vi "429 RT Driver Init.vi"(8 "error in":errorcluster, 11 "Device Reference in":T1 format="%.0x") -> (0 "error out":errorcluster, 1 "tx channel handle array":u32[](array[numeric]), 2 "rx channel handle array":u32[](array[numeric]), 3 "Device Reference out":T1 format="%.0x", 5 "board handle":u32)   [LabVIEW 2016, in "Ballard Arinc-429 Engine.lvlib"]
uses:
  Ballard Arinc-429 Engine.lvlib
  <vilib>/NI Veristand/Custom Device API/Custom Device Item Ref.ctl
  Shared/Controls and Global/Specify module by.ctl
  <instrlib>/AIT 429/Private/AIT 429 Initialize (SlotID).vi
  <instrlib>/AIT 429/Private/AIT 429 Initialize (Index).vi
  <instrlib>/AIT 429/Private/AIT 429 Initialize (Serial Number).vi
  <vilib>/NI Veristand/Custom Device API/Get Item Property (Variant).vi
  <vilib>/NI Veristand/Custom Device API/Get Item Property (U16).vi
  <vilib>/NI Veristand/Custom Device API/Get Item Property (Path).vi
  Shared/Controls and Global/Global.vi
  <vilib>/NI Veristand/Custom Device API/Custom Device API.lvlib
  Shared/Ballard Arinc-429 Shared.lvlib
  <instrlib>/AIT 429/AIT 429.lvlib
  <userlib>/ARINC-429/Owl429.lvlib
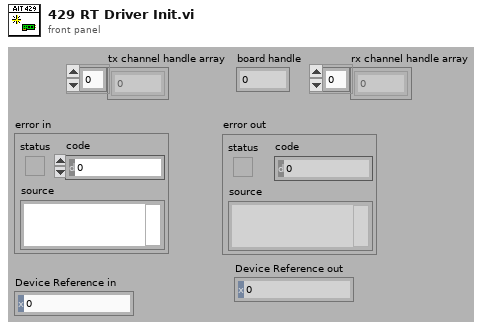
[diagram p1: front panel]
types:
  T1 = typedef "Custom Device API.lvlib/Custom Device Item Ref.ctl" = u64
  T2 = typedef "Ballard Arinc-429 Shared.lvlib/Specify module by.ctl" = enum16{"Index", "SlotID", "Serial number"}
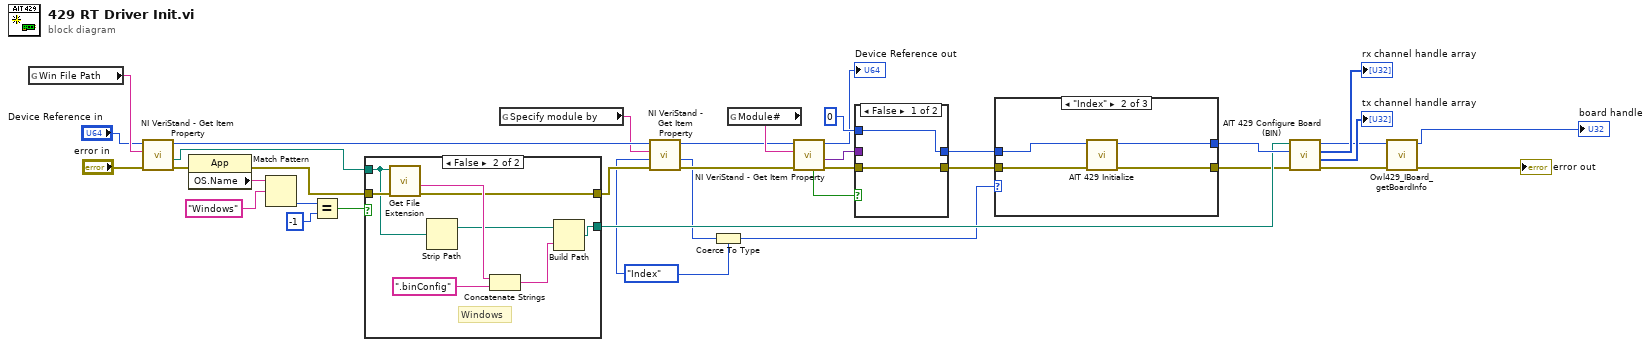
[diagram p0: block diagram]
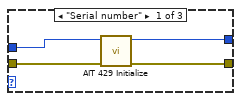
[diagram p2: hidden frame]
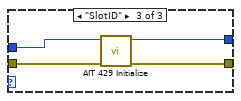
[diagram p3: hidden frame]
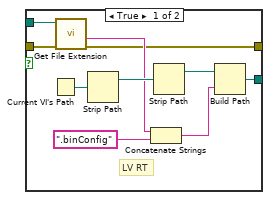
[diagram p4: hidden frame]
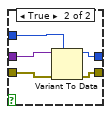
[diagram p5: hidden frame]
diagram:
  w3 = Specify_module_by."Index" ("Specify module by")
  n1 = global read "Global.vi" "Win File Path"() -> (w29:string)
  n2 = call-poly <vilib>:"NI VeriStand - Get Item Property.vi"("error in (no error)"="error in", "Property Name"=w29, "Item Ref in"="Device Reference in") -> ("error out"=w21:errorcluster, "Value"=w16:path, "Item Ref out"=w6:T1)  [unwired: 5 in, 1 out]
  n3 = property class="App"(error in=w21) -> (error out=w17:errorcluster, "OS.Name"=w10:string)  [unwired: 1 in, 1 out]
  n4 = Match Pattern(string=w10, regular expression="Windows") -> (offset past match=w19:i32)  [unwired: 1 in, 3 out]
  n5 = Equal?(x=w19, y=-1) -> (x = y?=w13:bool)
  n6 = case shown="False" w13 {
    tunnel: w17 -> [w37 w49]
    tunnel: w16 -> [w40 w48]
    tunnel: [w39 w51] -> w15
    tunnel: [w38 w50] -> w14
    frame True {
      # "LV RT"
      n7 = Current VI's Path() -> (path=w42:path)
      n8 = call <vilib>:"Get File Extension.vi"("error in (no error)"=w37, "file"=w40) -> ("error out"=w39:errorcluster, "filename without extension"=w41:string)  [unwired: 5 in, 3 out]
      n9 = Strip Path(path=w42) -> (stripped path=w43:path)  [unwired: 1 out]
      n10 = Concatenate Strings(w41, ".binConfig" ("string")) -> (w45:string)
      n11 = Strip Path(path=w43) -> (stripped path=w44:path)  [unwired: 1 out]
      n12 = Build Path(base path=w44, name or relative path=w45) -> (appended path=w38:path)
    }
    frame False {
      # "Windows"
      n13 = call <vilib>:"Get File Extension.vi"("error in (no error)"=w49, "file"=w48) -> ("error out"=w51:errorcluster, "filename without extension"=w52:string)  [unwired: 5 in, 3 out]
      n14 = Strip Path(path=w48) -> (stripped path=w47:path)  [unwired: 1 out]
      n15 = Concatenate Strings(w52, ".binConfig" ("string")) -> (w53:string)
      n16 = Build Path(base path=w47, name or relative path=w53) -> (appended path=w50:path)
    }
  }
  n17 = global read "Global.vi" "Specify module by"() -> (w4:string)
  n18 = call-poly <vilib>:"NI VeriStand - Get Item Property.vi"("error in (no error)"=w15, "Default Value"=w3, "Property Name"=w4, "Item Ref in"=w6) -> ("error out"=w7:errorcluster, "Value"=w2:u16, "Item Ref out"=w5:T1)  [unwired: 4 in, 1 out]
  n19 = Coerce To Type(0:w2, 1:w3) -> (2:w1:T2)
  n20 = global read "Global.vi" "Module#"() -> (w36:string)
  n21 = call-poly <vilib>:"NI VeriStand - Get Item Property.vi"("error in (no error)"=w7, "Property Name"=w36, "Item Ref in"=w5) -> ("error out"=w35:errorcluster, "Value"=w33:variant, "Item Ref out"=→"Device Reference out":T1, "Found?"=w34:bool)  [unwired: 5 in]
  n22 = case shown="False" w34 {
    tunnel: w35 -> [w55 w61]
    tunnel: w33 -> [_ w60]
    tunnel: u64 0 -> [w56 w59]
    tunnel: [w55 w58] -> w31
    tunnel: [w56 w57] -> w30
    frame False {
    }
    frame True {
      n23 = Variant To Data(error in=w61, type=w59, Variant=w60) -> (data=w57:u64, error out=w58:errorcluster)
    }
  }
  n24 = case shown="\"Index\"" w1 {
    tunnel: w31 -> [w65 w69 w73]
    tunnel: w30 -> [w64 w68 w72]
    tunnel: [w63 w67 w71] -> w28
    tunnel: [w62 w66 w70] -> w12
    frame "Serial number" {
      n25 = call-poly <instrlib>:"AIT 429 Initialize.vi"("error in (no error)"=w65, "serial number"=w64) -> ("error out"=w62:errorcluster, "board handle"=w63:u64)  [unwired: 8 in]
    }
    frame "Index" {
      n26 = call-poly <instrlib>:"AIT 429 Initialize.vi"("error in (no error)"=w69, "board index"=w68) -> ("error out"=w66:errorcluster, "board handle"=w67:u64)  [unwired: 8 in]
    }
    frame "SlotID" {
      n27 = call-poly <instrlib>:"AIT 429 Initialize.vi"("error in (no error)"=w73, "slot ID"=w72) -> ("error out"=w70:errorcluster, "board handle"=w71:u64)  [unwired: 8 in]
    }
  }
  n28 = call <instrlib>:"AIT 429 Configure Board (BIN).vi"("error in"=w12, "board handle"=w28, "Binary File path"=w14) -> ("error out"=w11:errorcluster, "tx channel handle array"=→"tx channel handle array":u64[], "rx channel handle array"=→"rx channel handle array":u64[], "board handle"=w24:u64)  [unwired: 3 in]
  n29 = call <userlib>:"Owl429_IBoard_getBoardInfo.vi"("error in (no error)"=w11, "board handle"=w24) -> ("error out"=→"error out":errorcluster, "board handle"=→"board handle":u64)  [unwired: 7 in, 1 out]
